vi "TCP-Send PXI Error.vi"(0 "connection ID":refnum<k5>, 11 "error in (no error)":errorcluster) -> (15 "error out":errorcluster)   [LabVIEW 2015]
uses:
  DAQ Engine VIs/PXI Globals.vi
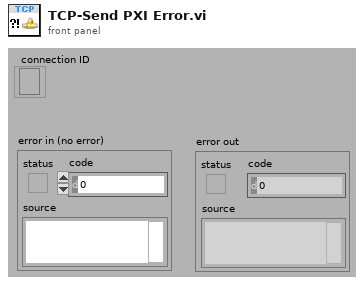
[diagram p1: front panel]
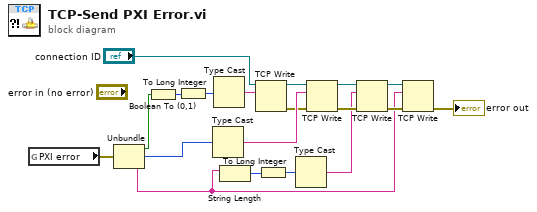
[diagram p0: block diagram]
diagram:
  n1 = global read "PXI Globals.vi" "PXI error"() -> (w18:errorcluster)
  n2 = Unbundle(w18) -> ("status"=w17:bool, "code"=w14:i32, "source"=w6:string)
  n3 = Boolean To (0,1)(Boolean=w17) -> (0, 1=w16:i16)
  n4 = To Long Integer(number=w16) -> (32bit integer=w15:i32)
  n5 = Type Cast(x=w14) -> (*(type *) &x=w13:string)  [unwired: 1 in]
  n6 = Type Cast(x=w15) -> (*(type *) &x=w19:string)  [unwired: 1 in]
  n7 = String Length(string=w6) -> (length=w5:i32)
  n8 = TCP Write(connection ID="connection ID", data in=w19) -> (connection ID out=w11:refnum<k5>, error out=w12:errorcluster)  [unwired: 2 in, 1 out]
  n9 = To Long Integer(number=w5) -> (32bit integer=w4:i32)
  n10 = Type Cast(x=w4) -> (*(type *) &x=w3:string)  [unwired: 1 in]
  n11 = TCP Write(connection ID=w11, data in=w13, error in (no error)=w12) -> (connection ID out=w10:refnum<k5>, error out=w8:errorcluster)  [unwired: 1 in, 1 out]
  n12 = TCP Write(connection ID=w10, data in=w3, error in (no error)=w8) -> (connection ID out=w9:refnum<k5>, error out=w7:errorcluster)  [unwired: 1 in, 1 out]
  n13 = TCP Write(connection ID=w9, data in=w6, error in (no error)=w7) -> (error out=→"error out":errorcluster)  [unwired: 1 in, 2 out]
